vi "Logging Equals - Entry.vi"(1 "Entry A":T1, 2 "Entry B":T1) -> (5 "Equal":bool)   [LabVIEW 2012, in "femtoRoboLib.lvlib"]
uses:
  femtoRoboLib.lvlib
  Controls/Log Entry.ctl
  Controls/Log Value Type.ctl
  Controls/Log Value Cluster.ctl
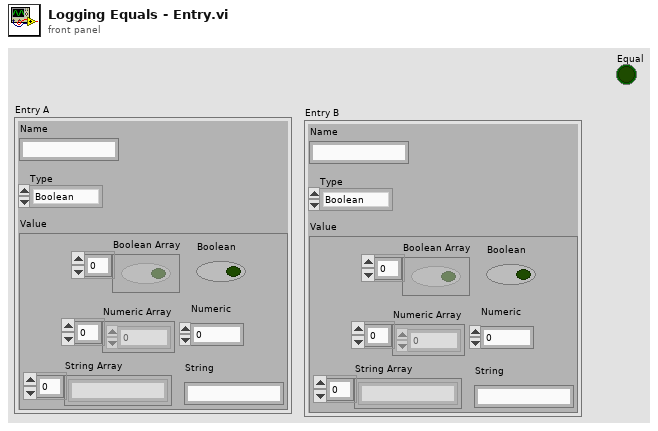
[diagram p1: front panel]
types:
  T1 = typedef "femtoRoboLib.lvlib/Log Entry.ctl" = cluster{"Name":string, "Type":T2, "Value":T3}
  T2 = typedef "femtoRoboLib.lvlib/Log Value Type.ctl" = enum16{"Boolean", "Numeric", "String", "Boolean Array", "Numeric Array", "String Array"}
  T3 = typedef "femtoRoboLib.lvlib/Log Value Cluster.ctl" = cluster{"Boolean Array":bool[], "Boolean":bool, "Numeric Array":dbl[], "Numeric":dbl, "String Array":string[], "String":string}
  T4 = typedef "femtoRoboLib.lvlib/Log Entry - Converted.ctl" = cluster{"Name":string, "Type":enum16{"Boolean", "Numeric", "String", "Boolean Array", "Numeric Array", "String Array"}, "Value":string, "ID":u32}
  T5 = cluster{"Name":bool, "Type":bool, "Value":bool, "ID":bool}
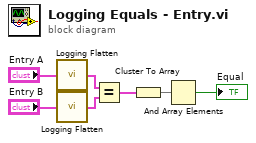
[diagram p0: block diagram]
diagram:
  n1 = call "Logging Flatten.vi"("In"="Entry A") -> ("Out"=w7:T4)
  n2 = call "Logging Flatten.vi"("In"="Entry B") -> ("Out"=w6:T4)
  n3 = Equal?(x=w7, y=w6) -> (x = y?=w5:T5)
  n4 = Cluster To Array(cluster=w5) -> (array=w4:bool[])
  n5 = And Array Elements(Boolean array=w4) -> (logical AND=→"Equal":bool)
